vi "随机数出数.vi"(6 "信号值原始值":dbl, 7 "公式":cluster{"X^2":dbl, "X":dbl, "B":dbl}={"X^2"=0.0, "X"=1.0, "B"=0.0}, 8 "启用":bool, 9 "采样值":dbl[](array[numeric]), 10 "参数输入":T1={"采样模式"=enum."自动采样", "采样点数"=3, "变异系数设定值"=0.1, "重新取值百分比"=0.5, "偏差模式"=enum."相对偏差", "相对偏差百分比"=0.0, "绝对偏差值"=0.0}, 11 "监测值原始值":dbl) -> (1 "采样值输出":dbl[](array[numeric]), 2 "参数输出":cluster{"mean":dbl, "变异系数":dbl, "随机数？":bool} {"mean" format="%0.2f"}, 3 "取值输出":dbl, 4 "信号值":dbl)   [LabVIEW 2016, in "random number.lvlib"]
uses:
  random number.lvlib
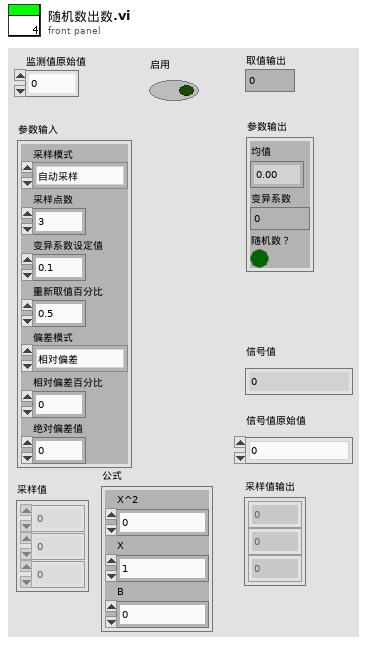
[diagram p1: front panel]
types:
  T1 = cluster{"采样模式":enum16{"自动采样", "手动采样"}, "采样点数":i32, "变异系数设定值":dbl, "重新取值百分比":dbl, "偏差模式":enum16{"相对偏差", "绝对偏差"}, "相对偏差百分比":dbl, "绝对偏差值":dbl}
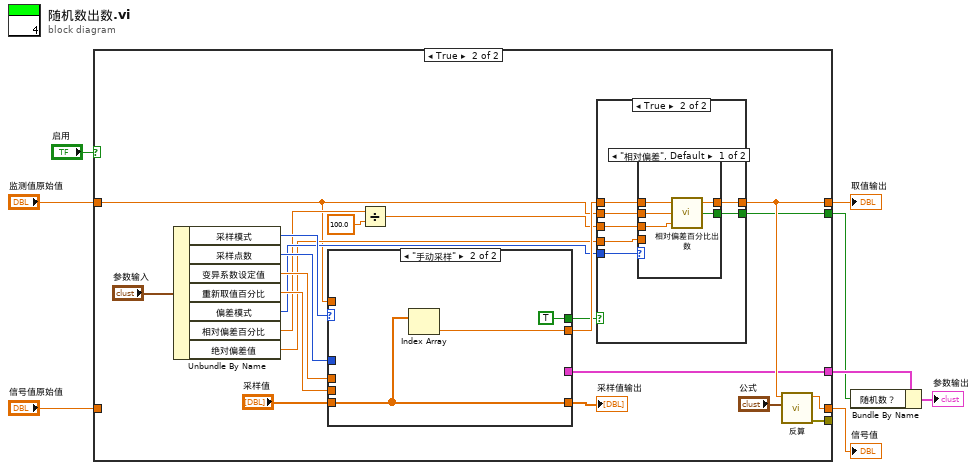
[diagram p0: block diagram]
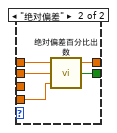
[diagram p4: hidden frame]
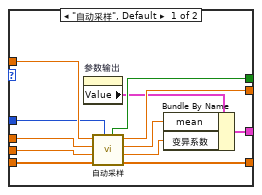
[diagram p5: hidden frame]
diagram:
  n1 = case shown="True" "启用" {
    tunnel: "监测值原始值" -> [w10 w16]
    tunnel: [w10 w20] -> w7
    tunnel: [_ w18] -> _
    tunnel: "信号值原始值" -> [w9 _]
    tunnel: [w9 w17] -> w4
    tunnel: [_ w15] -> w1
    tunnel: [_ w14] -> w3
    frame False {
    }
    frame True {
      n2 = Unbundle By Name("参数输入") -> ("采样模式"=w28:enum16{"自动采样", "手动采样"}, "采样点数"=w27:i32, "变异系数设定值"=w26:dbl, "重新取值百分比"=w25:dbl, "偏差模式"=w24:enum16{"相对偏差", "绝对偏差"}, "相对偏差百分比"=w23:dbl, "绝对偏差值"=w22:dbl)
      n3 = case shown="\"手动采样\"" w28 {
        tunnel: [w61 w63] -> w31
        tunnel: w16 -> [w60 _]
        tunnel: [w59 TRUE ("采样OK")] -> w30
        tunnel: w27 -> [w58 _]
        tunnel: w26 -> [w57 _]
        tunnel: w25 -> [w56 _]
        tunnel: "采样值" -> [w52 w62]
        tunnel: [w51 _] -> w14
        tunnel: [w50 w62] -> w13
        frame "自动采样", Default {
          n4 = property on="参数输出" class="Clust (strict)"() -> ("Value"=w55:cluster{"mean":dbl, "变异系数":dbl, "随机数？":bool})  [unwired: 2 in, 2 out]
          n5 = call "自动采样.vi"("采样点数"=w58, "采样值"=w52, "重新取值百分比"=w56, "变异系数设定值"=w57, "原始值"=w60) -> ("采样值输出"=w50:dbl[], "变异系数"=w53:dbl, "mean"=w54:dbl, "取值输出"=w61:dbl, "采样OK"=w59:bool)  [unwired: 2 in]
          n6 = Bundle By Name(cluster=w55, "mean"=w54, "变异系数"=w53) -> (w51:cluster{"mean":dbl, "变异系数":dbl, "随机数？":bool})
        }
        frame "手动采样" {
          n7 = Index Array(array=w62) -> (element=w63:dbl)  [unwired: 1 in]
        }
      }
      "采样值输出" <- w13
      n8 = Divide(x=w23, y=100.0) -> (x/y=w12:dbl)
      n9 = case shown="True" w30 {
        tunnel: w31 -> [w32 w39]
        tunnel: [w32 w38] -> w20
        tunnel: w24 -> [_ w37]
        tunnel: w12 -> [_ w36]
        tunnel: w22 -> [_ w35]
        tunnel: w16 -> [_ w34]
        tunnel: [_ w33] -> w15
        frame False {
        }
        frame True {
          n10 = case shown="\"相对偏差\", Default" w37 {
            tunnel: w39 -> [w44 w49]
            tunnel: [w43 w48] -> w38
            tunnel: w36 -> [w42 _]
            tunnel: w35 -> [_ w47]
            tunnel: w34 -> [w41 w45]
            tunnel: [w40 w46] -> w33
            frame "相对偏差", Default {
              n11 = call "相对偏差百分比出数.vi"("基准值"=w44, "原始值"=w41, "相对偏差百分比"=w42) -> ("取值输出"=w43:dbl, "随机数？"=w40:bool)  [unwired: 5 in]
            }
            frame "绝对偏差" {
              n12 = call "绝对偏差百分比出数.vi"("基准值"=w49, "原始值"=w45, "绝对偏差值"=w47) -> ("取值输出"=w48:dbl, "随机值？"=w46:bool)  [unwired: 5 in]
            }
          }
        }
      }
      n13 = call "反算.vi"("公式"="公式", "监测值"=w20) -> ("error out"=w18:errorcluster, "信号值"=w17:dbl)  [unwired: 8 in]
    }
  }
  "取值输出" <- w7
  "信号值" <- w4
  n14 = Bundle By Name(cluster=w3, "随机数？"=w1) -> (→"参数输出":cluster{"mean":dbl, "变异系数":dbl, "随机数？":bool})
